vi "Setup subWorker - gRPC Server.vi"(8 "error in":errorcluster, 11 "gRPC Server Tester in":refnum<class "gRPC Server Tester.lvclass">) -> (0 "error out":errorcluster, 3 "gRPC Server Tester out":refnum<class "gRPC Server Tester.lvclass">)   [LabVIEW 2019, in "gRPC Server Tester.lvclass"]
doc: "This VI sets up the framework parameters of a statically-linked subWorker."
uses:
  gRPC Server Tester.lvclass
  gRPC Server/gRPC Server/gRPC Server.lvclass
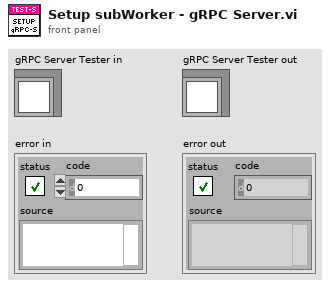
[diagram p1: front panel]
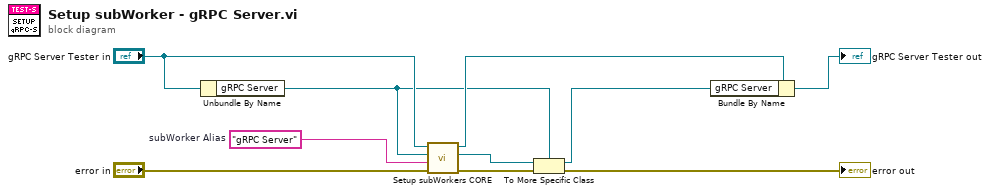
[diagram p0: block diagram]
diagram:
  w6 = "gRPC Server"  # subWorker Alias
  n1 = Unbundle By Name("gRPC Server Tester in") -> ("gRPC Server"=w3:refnum<class "gRPC Server.lvclass">)
  n2 = call-dynamic "Setup subWorkers CORE.vi"("error in"="error in", "subWorker Alias"=w6, "subWorker"=w3, "Worker"="gRPC Server Tester in") -> ("error out"=w5:errorcluster, "subWorker out"=w1:refnum<class "Worker.lvclass">, "Worker out"=w8:refnum<class "gRPC Server Tester.lvclass">)  [unwired: 5 in]
  n3 = To More Specific Class(target class=w3, reference=w1, error in=w5) -> (specific class reference=w2:refnum<class "gRPC Server.lvclass">, error out=→"error out":errorcluster)
  n4 = Bundle By Name(cluster=w8, "gRPC Server"=w2) -> (→"gRPC Server Tester out":refnum<class "gRPC Server Tester.lvclass">)
